vi "SLSC Update Default Values in Tree.vi"(8 "error in (no error)":errorcluster, 10 "SLSC Output Tree":T1(array[cluster]), 11 "SLSC EDS module in":T2) -> (0 "error out":errorcluster, 3 "SLSC EDS module out":T2)   [LabVIEW 2015, in "SLSC EDS System Explorer.lvlib"]
uses:
  SLSC EDS System Explorer.lvlib
  SLSC EDS API/JSON parsing/EDSjsonStructure.ctl
  SLSC EDS API/JSON parsing/enum.ctl
  SLSC EDS API/JSON parsing/property.ctl
  SLSC EDS API/JSON parsing/command.ctl
  SLSC EDS API/JSON parsing/scale.ctl
  SLSC EDS API/JSON parsing/physicalChannel.ctl
  SLSC EDS API/JSON parsing/register.ctl
  SLSC UI API/SLSC Tree Control.lvlib
panel:
  # "not working\nregisterMap->registers->initialValue"
  # "not working\nregisterMap->registers->initialValue"
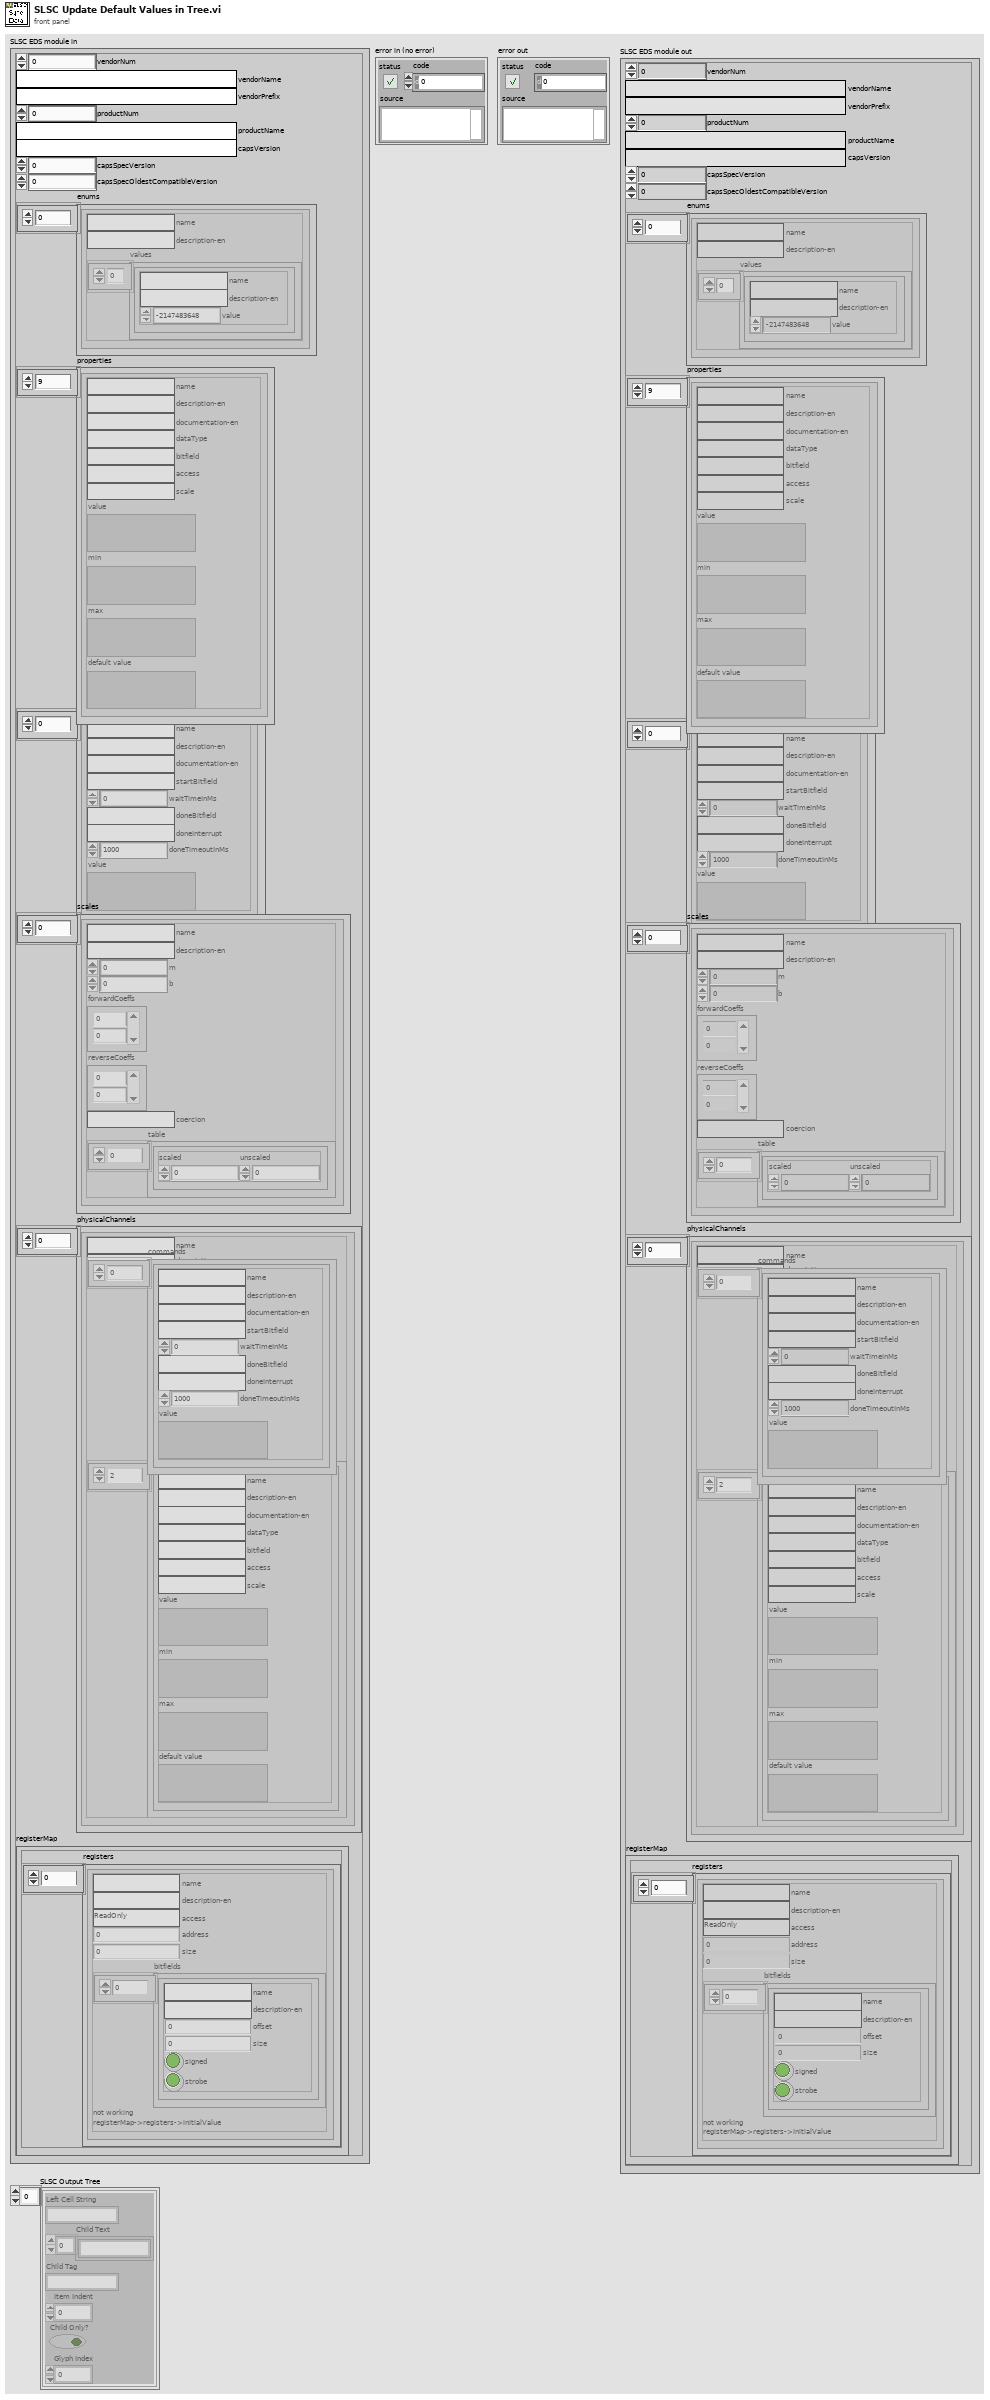
[diagram p1: front panel]
types:
  T1 = cluster{"Left Cell String":string, "Child Text":string[], "Child Tag":string, "Item Indent":i32, "Child Only?":bool, "Glyph Index":i32}[]
  T2 = typedef "EDSjsonStructure.ctl" = cluster{"vendorNum":u32, "vendorName":string, "vendorPrefix":string, "productNum":u32, "productName":string, "capsVersion":string, "capsSpecVersion":u32, "capsSpecOldestCompatibleVersion":u32, "enums":T3[], "properties":T4[], "commands":T5[], "scales":T6[], "physicalChannels":T7[], "registerMap":cluster{"registers":T8[]}}
  T3 = typedef "enum.ctl" = cluster{"name":string, "description-en":string, "values":cluster{"name":string, "description-en":string, "value":i32}[]}
  T4 = typedef "property.ctl" = cluster{"name":string, "description-en":string, "documentation-en":string, "dataType":string, "bitfield":string, "access":string, "scale":string, "value":variant, "min":variant, "max":variant, "default value":variant}
  T5 = typedef "command.ctl" = cluster{"name":string, "description-en":string, "documentation-en":string, "startBitfield":string, "waitTimeInMs":i32, "doneBitfield":string, "doneInterrupt":string, "doneTimeoutInMs":i32, "value":variant}
  T6 = typedef "scale.ctl" = cluster{"name":string, "description-en":string, "m":dbl, "b":dbl, "forwardCoeffs":dbl[], "reverseCoeffs":dbl[], "coercion":string, "table":cluster{"scaled":dbl, "unscaled":dbl}[]}
  T7 = typedef "physicalChannel.ctl" = cluster{"name":string, "description-en":string, "commands":T5[], "properties":T4[]}
  T8 = typedef "register.ctl" = cluster{"name":string, "description-en":string, "access":string, "address":u32, "size":u32, "bitfields":cluster{"name":string, "description-en":string, "offset":u32, "size":u32, "signed":bool, "strobe":bool}[]}
  T9 = cluster{"Left Cell String":string, "Child Text":string[], "Child Tag":string, "Item Indent":i32, "Child Only?":bool, "Glyph Index":i32}
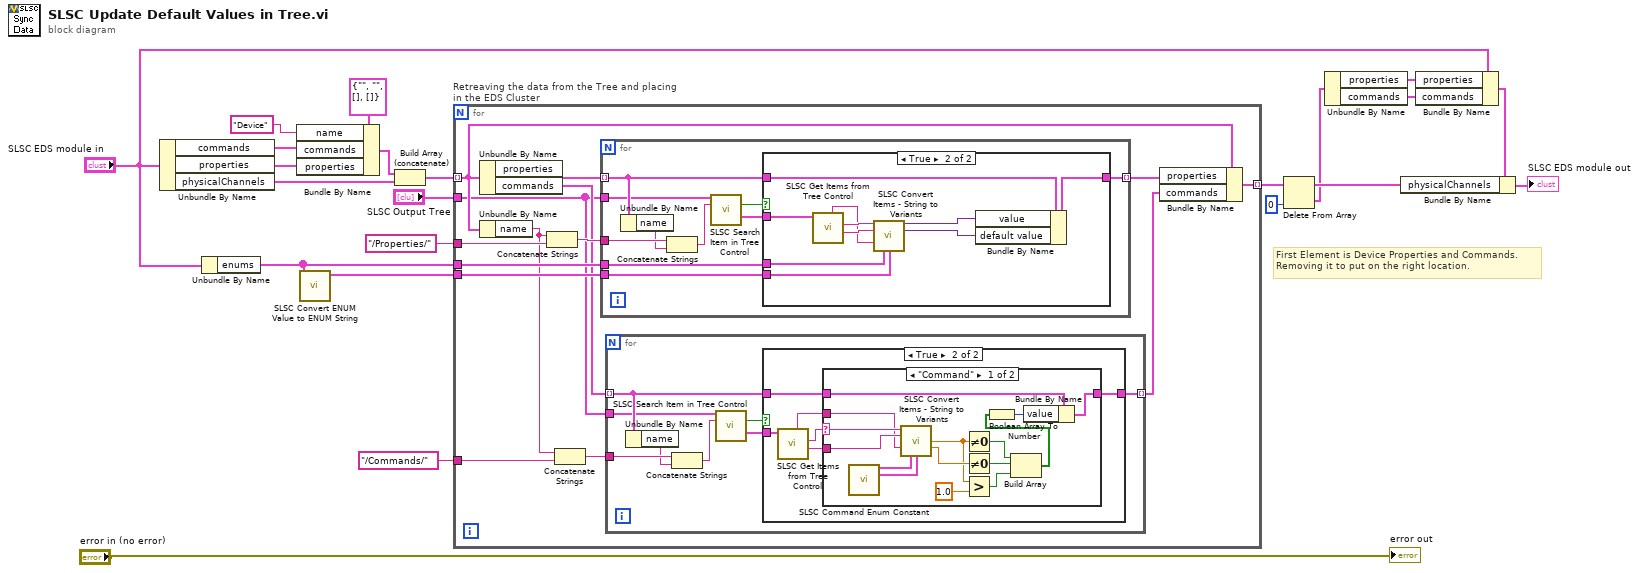
[diagram p0: block diagram]
diagram:
  # "First Element is Device Properties and Commands.\nRemoving it to put on the right location."
  n1 = Unbundle By Name("SLSC EDS module in") -> ("commands"=w3:T5[], "properties"=w9:T4[], "physicalChannels"=w2:T7[])
  n2 = Unbundle By Name("SLSC EDS module in") -> ("enums"=w20:T3[])
  n3 = Bundle By Name(cluster=T7 {"name"="", "description-en"="", "commands"=[], "properties"=[]} ("physicalChannel"), "name"="Device", "commands"=w3, "properties"=w9) -> (w8:T7)
  n4 = call "SLSC Convert ENUM Value to ENUM String.vi"("Enums"=w20) -> ("String Enums"=w21:cluster{"name":string, "string enums":string}[])  [unwired: 9 in, 1 out]
  n5 = Build Array (concatenate)(w8, w2) -> (w14:T7[])
  n6 = for "Retreaving the data from the Tree and placing in the EDS Cluster" {
    tunnel: w14 -> [w26] mode=indexing
    tunnel: "SLSC Output Tree" -> [w23]
    tunnel: w21 -> [w35]
    tunnel: w20 -> [w34]
    tunnel: "/Properties/" ("name") -> [w33]
    tunnel: [w30] -> w11 mode=indexing
    tunnel: "/Commands/" ("name") -> [w27]
    n7 = Unbundle By Name(w26) -> ("properties"=w36:T4[], "commands"=w29:T5[])
    n8 = Unbundle By Name(w26) -> ("name"=w25:string)
    n9 = Concatenate Strings(w25, w33) -> (w32:string)
    n10 = Concatenate Strings(w25, w27) -> (w28:string)
    n11 = for {
      tunnel: w23 -> [w68]
      tunnel: w36 -> [w72] mode=indexing
      tunnel: w32 -> [w76]
      tunnel: [w71] -> w31 mode=indexing
      tunnel: w34 -> [w73]
      tunnel: w35 -> [w70]
      n12 = Unbundle By Name(w72) -> ("name"=w75:string)
      n13 = Concatenate Strings(w76, w75) -> (w74:string)
      n14 = call "SLSC Search Item in Tree Control.vi"("SLSC Output Tree"=w68, "Item Tag"=w74) -> ("Found?"=w69:bool, "Item"=w77:T9)  [unwired: 10 in, 2 out]
      n15 = case shown="True" w69 {
        tunnel: w77 -> [_ w88]
        tunnel: w73 -> [_ w86]
        tunnel: w72 -> [w78 w87]
        tunnel: [w78 w85] -> w71
        tunnel: w70 -> [_ w82]
        frame False {
        }
        frame True {
          n16 = call "SLSC Get Items from Tree Control.vi"("Item"=w88) -> ("Value"=w80:string, "Datatype"=w81:string, "Reset Value"=w79:string)  [unwired: 6 in, 2 out]
          n17 = call "SLSC Convert Items - String to Variants.vi"("Datatype"=w81, "Value"=w80, "Reset Value"=w79, "enums"=w86, "string enums"=w82) -> ("Value"=w84:variant, "Reset Value"=w83:variant)  [unwired: 7 in, 2 out]
          n18 = Bundle By Name(cluster=w87, "value"=w84, "default value"=w83) -> (w85:T4)
        }
      }
    }
    n19 = for {
      tunnel: w23 -> [w37]
      tunnel: w29 -> [w40] mode=indexing
      tunnel: w28 -> [w43]
      tunnel: [w39] -> w24 mode=indexing
      n20 = Unbundle By Name(w40) -> ("name"=w42:string)
      n21 = Concatenate Strings(w43, w42) -> (w41:string)
      n22 = call "SLSC Search Item in Tree Control.vi"("SLSC Output Tree"=w37, "Item Tag"=w41) -> ("Found?"=w38:bool, "Item"=w44:T9)  [unwired: 10 in, 2 out]
      n23 = case shown="True" w38 {
        tunnel: w44 -> [_ w51]
        tunnel: w40 -> [w45 w49]
        tunnel: [w45 w46] -> w39
        frame False {
        }
        frame True {
          n24 = call "SLSC Get Items from Tree Control.vi"("Item"=w51) -> ("Value"=w48:string, "Datatype"=w50:string, "Reset Value"=w47:string)  [unwired: 6 in, 2 out]
          n25 = case shown="\"Command\"" w50 {
            selector: w50 -> [w62 _]
            tunnel: w48 -> [w61 _]
            tunnel: w49 -> [w65 w67]
            tunnel: [w66 w67] -> w46
            tunnel: w47 -> [w58 _]
            frame "Command" {
              n26 = call "SLSC Command Enum Constant.vi"() -> ("Array"=w60:T3[], "String Enums"=w59:cluster{"name":string, "string enums":string}[])  [unwired: 11 in, 3 out]
              n27 = call "SLSC Convert Items - String to Variants.vi"("Datatype"=w62, "Value"=w61, "Reset Value"=w58, "enums"=w60, "string enums"=w59) -> ("Value (DBL)"=w54:dbl, "Reset Value (DBL)"=w57:dbl)  [unwired: 7 in, 2 out]
              n28 = Not Equal To 0?(x=w54) -> (x != 0?=w56:bool)
              n29 = Not Equal To 0?(x=w57) -> (x != 0?=w55:bool)
              n30 = Greater?(x=w54, y=1.0) -> (0:w52:bool)
              n31 = Build Array(w56, w55, w52) -> (w64:bool[])
              n32 = Boolean Array To Number(Boolean array=w64) -> (number=w63:u32)
              n33 = Bundle By Name(cluster=w65, "value"=w63) -> (w66:T5)
            }
            frame Default {
            }
          }
        }
      }
    }
    n34 = Bundle By Name(cluster=w26, "properties"=w31, "commands"=w24) -> (w30:T7)
  }
  n35 = Delete From Array(array=w11, index=0) -> (deleted portion=w7:T7, array with subset deleted=w13:T7[])  [unwired: 1 in]
  n36 = Unbundle By Name(w7) -> ("properties"=w6:T4[], "commands"=w5:T5[])
  n37 = Bundle By Name(cluster="SLSC EDS module in", "properties"=w6, "commands"=w5) -> (w18:T2)
  n38 = Bundle By Name(cluster=w18, "physicalChannels"=w13) -> (→"SLSC EDS module out":T2)
  "error out" <- "error in (no error)"
